vi "From Float Tree Data.vi"(11 "Tree Data":refnum<class "Tree Data.lvclass">) -> (2 "Float":dbl)   [LabVIEW 2020, in "NI_VIAnCFGDataStructure.lvlib" / "Flt.lvclass"]
doc: "Extract a Float value from Tree Data type."
uses:
  <vilib>/addons/analyzer/VIAnCFGDataStructure/Data Types/Float/Flt.lvclass
  <vilib>/addons/analyzer/VIAnCFGDataStructure/Tree Data/Tree Data.lvclass
  <vilib>/addons/analyzer/VIAnCFGDataStructure/Data Types/Float/Flt.lvclass/Flt.ctl
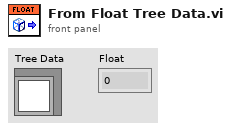
[diagram p1: front panel]
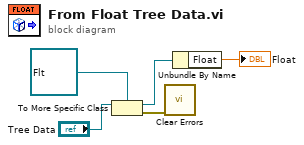
[diagram p0: block diagram]
diagram:
  n1 = To More Specific Class(target class=refnum<class "Flt.lvclass"> refnum ("Float.lvclass"), reference="Tree Data") -> (specific class reference=w4:refnum<class "Flt.lvclass">, error out=w3:errorcluster)  [unwired: 1 in]
  n2 = call <vilib>:"Clear Errors.vi"("error in (no error)"=w3) -> ()  [unwired: 5 in, 2 out]
  n3 = Unbundle By Name(w4) -> ("Float"=→"Float":dbl)
